vi "Loop_Auto.vi"() -> ()   [LabVIEW 2017, in "Autonomous.lvlib"]
uses:
  Autonomous.lvlib
  ENUM_Auto_State.ctl
  TypeDef/CLUSTER_CMD_WC_Drive.ctl
  TypeDef/ENUM_WC_Drive_DriveMode.ctl
  TypeDef/CLUSTER_Drive_ACT Loop_VBus Data.ctl
  TypeDef/CLUSTER_X and Y.ctl
  TypeDef/CLUSTER_Drive_ACT Loop_Profile Data.ctl
  <vilib>/Rock Robotics/WPI/ThirdParty/Sensors/navX/_TypeDefs/FRIC_navX_DeviceNumbersTypeDef.ctl
  ENUM_Auto_Action.ctl
  _SHARE ALL/Global Share All/Global_STOP.vi
  WC_Drive/Global_WC_Drive_Encoder_Values.vi
  Globals/Global_CMD_Drive.vi
panel:
  out "Cycle Time (S)":dbl format="%.3g"
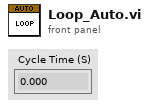
[diagram p1: front panel]
types:
  T1 = typedef "CLUSTER_CMD_WC_Drive.ctl" = cluster{"Drive_Mode":T2, "VBus":T3, "Profile":T5, "Zero Drive Encoders":bool, "Set Target Position(IN)":dbl, "Target Angle(Degree)":dbl, "Lock Angle":bool, "Zero YAW":bool}
  T2 = typedef "ENUM_WC_Drive_DriveMode.ctl" = enum16{"Motion Profile", "CrossLineAuto", "VBus", "Stop"}
  T3 = typedef "CLUSTER_Drive_ACT Loop_VBus Data.ctl" = cluster{"Drive":T4, "Turbo":bool}
  T4 = typedef "CLUSTER_X and Y.ctl" = cluster{"Steer":dbl, "Throtle":dbl}
  T5 = typedef "CLUSTER_Drive_ACT Loop_Profile Data.ctl" = cluster{"Start":bool}
  T6 = typedef "Autonomous.lvlib/ENUM_Auto_State.ctl" = enum16{"Startup", "Idle", "Rotate 180", "Cross Line", "Shutdown"}
  T7 = typedef "Autonomous.lvlib/ENUM_Auto_Action.ctl" = enum16{"No Action", "Reset Time", "Reset All", "Lock Angle", "Drive", "Zero Drive Encoders", "Zero YAW"}
  T8 = cluster{"State":T6, "Previous State":T6, "Current Time":timestamp, "Previous Time":timestamp, "Start Time":timestamp, "Target Time (ms)":u32, "Cycle Time(S)":dbl, "CMD_Drive_Data":T1, "Test":dbl, "Steering":dbl, "Throtal":dbl, "Encoder Target Position(in)":dbl, "Zero Drive Encoders":bool, "Lock Angle":bool, "Target Angle(Degree)":dbl, "Zero YAW":bool, "Left Encoder":i32, "Right Encoder":i32, "YAW":dbl}
  T9 = typedef "FRIC_navX_DeviceNumbersTypeDef.ctl" = enum16{"Dev0", "Dev1", "Dev2", "Dev3"}
  T10 = cluster{"Rollover":dbl, "Yaw":dbl, "Cont Yaw":dbl}
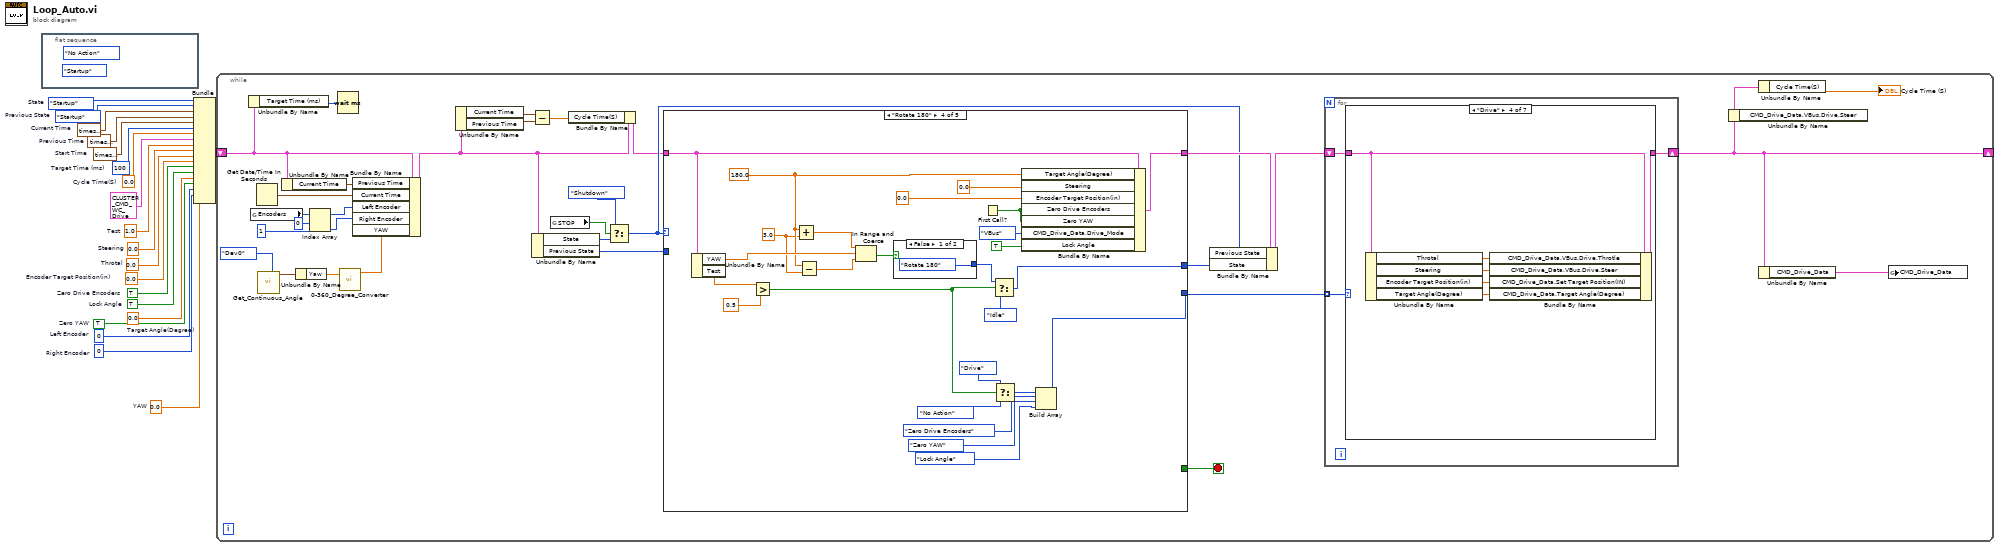
[diagram p0: block diagram]
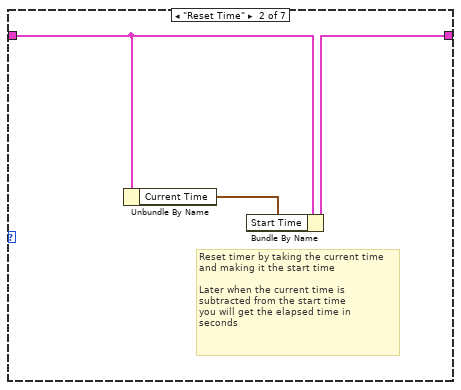
[diagram p3: hidden frame]
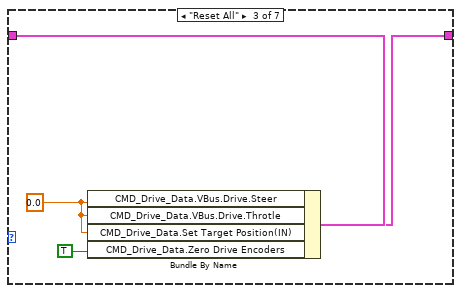
[diagram p4: hidden frame]
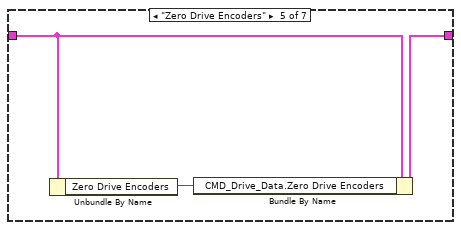
[diagram p5: hidden frame]
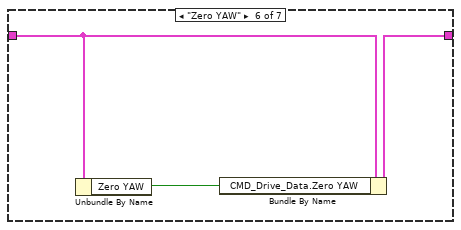
[diagram p6: hidden frame]
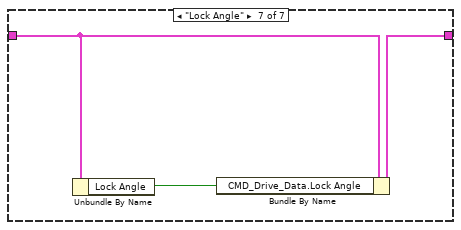
[diagram p7: hidden frame]
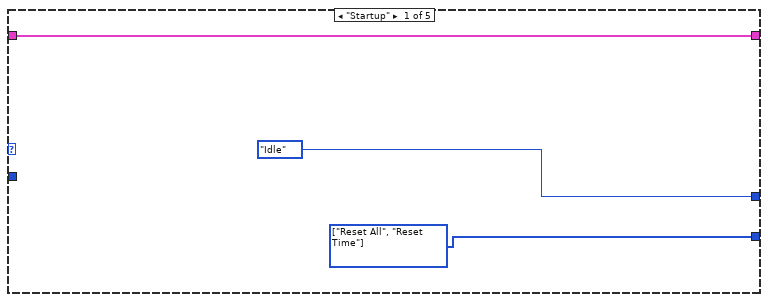
[diagram p8: hidden frame]
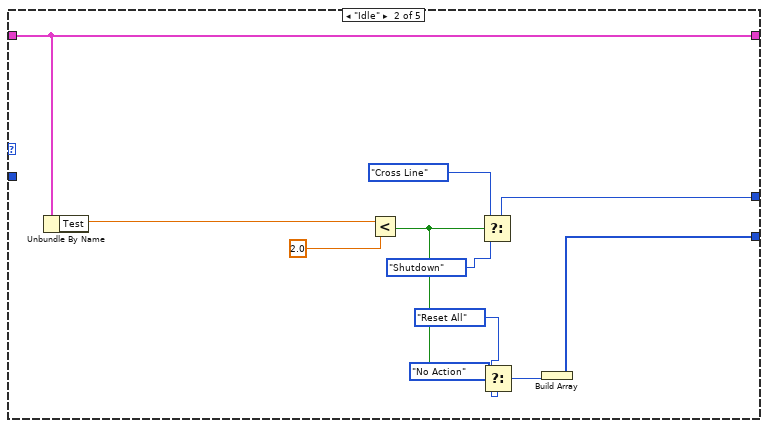
[diagram p9: hidden frame]
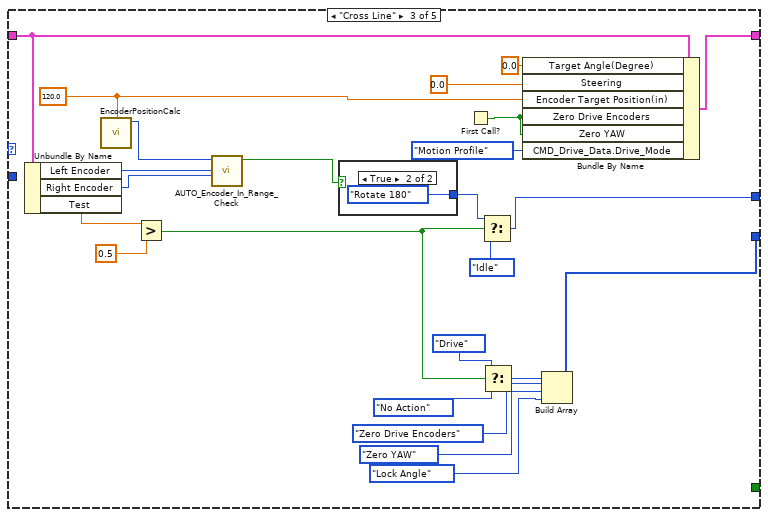
[diagram p10: hidden frame]
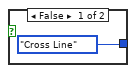
[diagram p11: hidden frame]
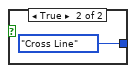
[diagram p12: hidden frame]
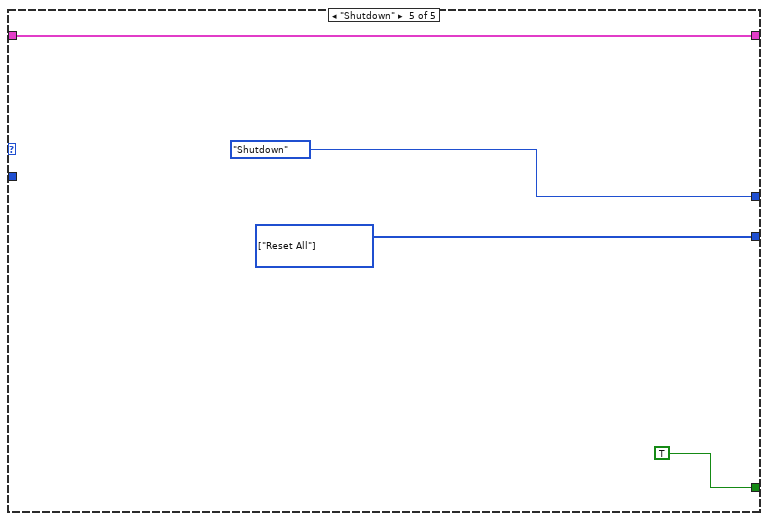
[diagram p13: hidden frame]
diagram:
  w1 = 0.0  # YAW
  w2 = 0  # Right Encoder
  w3 = 0  # Left Encoder
  w4 = TRUE  # Zero YAW
  w5 = 0.0  # Target Angle(Degree)
  w6 = TRUE  # Lock Angle
  w7 = TRUE  # Zero Drive Encoders
  w8 = 0.0  # Encoder Target Position(in)
  w9 = 0.0  # Throtal
  w10 = 0.0  # Steering
  w11 = 1.0  # Test
  w13 = 0.0  # Cycle Time(S)
  w14 = ENUM_Auto_State."Startup"  # Previous State
  w15 = timestamp(0 s since 1904-01-01)  # Previous Time
  w16 = u32 100  # Target Time (ms)
  w17 = timestamp(0 s since 1904-01-01)  # Start Time
  w18 = timestamp(0 s since 1904-01-01)  # Current Time
  w19 = ENUM_Auto_State."Startup"  # State
  n1 = flat-sequence {
    frame #0 {
      (unwired) ENUM_Auto_State."Startup" ("State")
      (unwired) ENUM_Auto_Action."No Action" ("Action")
    }
  }
  n2 = Bundle("State"=w19, "Previous State"=w14, "Current Time"=w18, "Previous Time"=w15, "Start Time"=w17, "Target Time (ms)"=w16, "Cycle Time(S)"=w13, "CMD_Drive_Data"=T1 {"Drive_Mode"=enum."Motion Profile", "VBus"={"Drive"={"Steer"=0.0, "Throtle"=0.0}, "Turbo"=FALSE}, "Profile"={"Start"=FALSE}, "Zero Drive Encoders"=FALSE, "Set Target Position(IN)"=0.0, "Target Angle(Degree)"=0.0, "Lock Angle"=FALSE, "Zero YAW"=FALSE}, "Test"=w11, "Steering"=w10, "Throtal"=w9, "Encoder Target Position(in)"=w8, "Zero Drive Encoders"=w7, "Lock Angle"=w6, "Target Angle(Degree)"=w5, "Zero YAW"=w4, "Left Encoder"=w3, "Right Encoder"=w2, "YAW"=w1) -> (w20:T8)  [unwired: 1 in]
  n3 = while {
    shift-right: [w39] -> _
    shift-left: w20 -> [w42]
    stop <- w31 stop-if-true
    n4 = Unbundle By Name(w42) -> ("Target Time (ms)"=w44:u32)
    n5 = global read "Global_WC_Drive_Encoder_Values.vi" "Encoders"() -> (w29:i32[])
    n6 = Get Date/Time In Seconds() -> (seconds since 1Jan1904=w51:timestamp)
    n7 = call <vilib>:"Get_Continuous_Angle.vi"("Device Number"=FRIC_navX_DeviceNumbersTypeDef."Dev0") -> ("Continuous Angle"=w23:T10)  [unwired: 10 in]
    n8 = Unbundle By Name(w42) -> ("Current Time"=w43:timestamp)
    n9 = Unbundle By Name(w23) -> ("Yaw"=w22:dbl)
    n10 = Index Array(array=w29, index #1=0 ("index"), index #2=1 ("index")) -> (element #1=w28:i32, element #2=w27:i32)
    n11 = Wait (ms)(milliseconds to wait=w44) -> ()  [unwired: 1 out]
    n12 = call "0-360_Degree_Converter.vi"("Yaw in"=w22) -> ("Yaw out"=w21:dbl)  [unwired: 10 in]
    n13 = Bundle By Name(cluster=w42, "Previous Time"=w43, "Current Time"=w51, "Left Encoder"=w28, "Right Encoder"=w27, "YAW"=w21) -> (w35:T8)
    n14 = Unbundle By Name(w35) -> ("Current Time"=w36:timestamp, "Previous Time"=w37:timestamp)
    n15 = Subtract(x=w36, y=w37) -> (x-y=w33:dbl)
    n16 = Unbundle By Name(w35) -> ("State"=w45:T6, "Previous State"=w41:T6)
    n17 = global read "Global_STOP.vi" "STOP"() -> (w47:bool)
    n18 = Bundle By Name(cluster=w35, "Cycle Time(S)"=w33) -> (w34:T8)
    n19 = Select(t=ENUM_Auto_State."Shutdown" ("State"), s=w47, f=w45) -> (s? t:f=w40:T6)
    n20 = case shown="\"Rotate 180\"" w40 {
      tunnel: w34 -> [w80 w91 w106 w134 w149]
      tunnel: [w80 w91 w105 w133 w149] -> w49
      tunnel: [ENUM_Auto_State."Idle" ("State") w90 w115 w143 ENUM_Auto_State."Shutdown" ("State")] -> w48
      tunnel: [w79 w83 w109 w137 w147] -> w32
      tunnel: w41 -> [_ _ _ _ _]
      tunnel: [_ _ _ _ TRUE] -> w31
      frame "Startup" {
        w79 = T7[] [enum."Reset All", enum."Reset Time"] items=["No Action", "Reset Time", "Reset All", "Lock Angle", "Drive", "Zero Drive Encoders", "Zero YAW"] ("Actions")
      }
      frame "Idle" {
        n21 = Unbundle By Name(w91) -> ("Test"=w82:dbl)
        n22 = Less?(x=w82, y=2.0) -> (x < y?=w85:bool)
        n23 = Select(t=ENUM_Auto_State."Cross Line" ("State"), s=w85, f=ENUM_Auto_State."Shutdown" ("State")) -> (s? t:f=w90:T6)
        n24 = Select(t=ENUM_Auto_Action."Reset All" ("Action"), s=w85, f=ENUM_Auto_Action."No Action" ("Action")) -> (s? t:f=w84:T7)
        n25 = Build Array(w84) -> (w83:T7[])
      }
      frame "Cross Line" {
        w96 = 120.0 ("Encoder Target Position(in)")
        n26 = Unbundle By Name(w106) -> ("Left Encoder"=w94:i32, "Right Encoder"=w93:i32, "Test"=w108:dbl)
        n27 = call "EncoderPositionCalc.vi"("PositionTarget(in)"=w96) -> ("PostionTarget(Counts)"=w92:i32)  [unwired: 10 in]
        n28 = Greater?(x=w108, y=0.5) -> (0:w111:bool)
        n29 = call "AUTO_Encoder_In_Range_Check.vi"("Right Encoder"=w93, "Left Encoder"=w94, "PostionTarget(Counts)"=w92) -> ("Boolean"=w95:bool)  [unwired: 8 in]
        n30 = case shown="True" w95 {
          tunnel: [ENUM_Auto_State."Cross Line" ("State") ENUM_Auto_State."Rotate 180" ("State")] -> w97
          frame False {
          }
          frame True {
          }
        }
        n31 = First Call?() -> (First Call?: T/F=w101:bool)
        n32 = Select(t=w97, s=w111, f=ENUM_Auto_State."Idle" ("State")) -> (s? t:f=w115:T6)
        n33 = Select(t=ENUM_Auto_Action."Drive" ("Action"), s=w111, f=ENUM_Auto_Action."No Action" ("Action")) -> (s? t:f=w110:T7)
        n34 = Bundle By Name(cluster=w106, "Target Angle(Degree)"=0.0, "Steering"=0.0, "Encoder Target Position(in)"=w96, "Zero Drive Encoders"=w101, "Zero YAW"=w101, "CMD_Drive_Data.Drive_Mode"=ENUM_WC_Drive_DriveMode."Motion Profile") -> (w105:T8)
        n35 = Build Array(w110, ENUM_Auto_Action."Zero Drive Encoders" ("Action"), ENUM_Auto_Action."Zero YAW" ("Action"), ENUM_Auto_Action."Lock Angle" ("Action")) -> (w109:T7[])
      }
      frame "Rotate 180" {
        w119 = 3.0 ("y")
        w120 = 180.0 ("Target Angle(Degree)")
        n36 = Unbundle By Name(w134) -> ("YAW"=w123:dbl, "Test"=w136:dbl)
        n37 = Greater?(x=w136, y=0.5) -> (0:w139:bool)
        n38 = Add(x=w120, y=w119) -> (x+y=w122:dbl)
        n39 = Subtract(x=w120, y=w119) -> (x-y=w121:dbl)
        n40 = In Range and Coerce(upper limit=w122, x=w123, lower limit=w121) -> (In Range?=w124:bool)  [unwired: 1 out]
        n41 = case shown="False" w124 {
          tunnel: [ENUM_Auto_State."Rotate 180" ("State") ENUM_Auto_State."Cross Line" ("State")] -> w126
          frame False {
          }
          frame True {
          }
        }
        n42 = First Call?() -> (First Call?: T/F=w130:bool)
        n43 = Select(t=w126, s=w139, f=ENUM_Auto_State."Idle" ("State")) -> (s? t:f=w143:T6)
        n44 = Select(t=ENUM_Auto_Action."Drive" ("Action"), s=w139, f=ENUM_Auto_Action."No Action" ("Action")) -> (s? t:f=w138:T7)
        n45 = Bundle By Name(cluster=w134, "Target Angle(Degree)"=w120, "Steering"=0.0, "Encoder Target Position(in)"=0.0, "Zero Drive Encoders"=w130, "Zero YAW"=w130, "CMD_Drive_Data.Drive_Mode"=ENUM_WC_Drive_DriveMode."VBus", "Lock Angle"=TRUE) -> (w133:T8)
        n46 = Build Array(w138, ENUM_Auto_Action."Zero Drive Encoders" ("Action"), ENUM_Auto_Action."Zero YAW" ("Action"), ENUM_Auto_Action."Lock Angle" ("Action")) -> (w137:T7[])
      }
      frame "Shutdown" {
        w147 = T7[] [enum."Reset All"] items=["No Action", "Reset Time", "Reset All", "Lock Angle", "Drive", "Zero Drive Encoders", "Zero YAW"] ("Actions")
      }
    }
    n47 = Bundle By Name(cluster=w49, "Previous State"=w40, "State"=w48) -> (w50:T8)
    n48 = for {
      tunnel: w32 -> [w54] mode=indexing
      shift-right: [w53] -> w39
      shift-left: w50 -> [w52]
      n49 = case shown="\"Drive\"" w54 {
        tunnel: w52 -> [w55 w58 w62 w68 w71 w74 w77]
        tunnel: [w55 w57 w61 w67 w70 w73 w76] -> w53
        frame "No Action" {
        }
        frame "Reset Time" {
          # "Reset timer by taking the current time\nand making it the start time\n\nLater when the current time is \nsubtracted from the start time\nyou will get the elapsed time in \nseconds"
          n50 = Unbundle By Name(w58) -> ("Current Time"=w56:timestamp)
          n51 = Bundle By Name(cluster=w58, "Start Time"=w56) -> (w57:T8)
        }
        frame "Reset All" {
          w60 = 0.0 ("FG Write Value")
          n52 = Bundle By Name(cluster=w62, "CMD_Drive_Data.VBus.Drive.Steer"=w60, "CMD_Drive_Data.VBus.Drive.Throtle"=w60, "CMD_Drive_Data.Set Target Position(IN)"=w60, "CMD_Drive_Data.Zero Drive Encoders"=TRUE ("Output Bool")) -> (w61:T8)
        }
        frame "Drive" {
          n53 = Unbundle By Name(w68) -> ("Throtal"=w66:dbl, "Steering"=w65:dbl, "Encoder Target Position(in)"=w64:dbl, "Target Angle(Degree)"=w63:dbl)
          n54 = Bundle By Name(cluster=w68, "CMD_Drive_Data.VBus.Drive.Throtle"=w66, "CMD_Drive_Data.VBus.Drive.Steer"=w65, "CMD_Drive_Data.Set Target Position(IN)"=w64, "CMD_Drive_Data.Target Angle(Degree)"=w63) -> (w67:T8)
        }
        frame "Zero Drive Encoders" {
          n55 = Unbundle By Name(w71) -> ("Zero Drive Encoders"=w69:bool)
          n56 = Bundle By Name(cluster=w71, "CMD_Drive_Data.Zero Drive Encoders"=w69) -> (w70:T8)
        }
        frame "Zero YAW" {
          n57 = Unbundle By Name(w74) -> ("Zero YAW"=w72:bool)
          n58 = Bundle By Name(cluster=w74, "CMD_Drive_Data.Zero YAW"=w72) -> (w73:T8)
        }
        frame "Lock Angle" {
          n59 = Unbundle By Name(w77) -> ("Lock Angle"=w75:bool)
          n60 = Bundle By Name(cluster=w77, "CMD_Drive_Data.Lock Angle"=w75) -> (w76:T8)
        }
      }
    }
    n61 = Unbundle By Name(w39) -> ()  [unwired: 1 out]
    n62 = Unbundle By Name(w39) -> ("Cycle Time(S)"=→"Cycle Time (S)":dbl)
    n63 = Unbundle By Name(w39) -> ("CMD_Drive_Data"=w30:T1)
    n64 = global write "Global_CMD_Drive.vi" "CMD_Drive_Data"(w30) -> ()
  }
